vi "GE 1.vi"() -> ()   [LabVIEW 2014]
uses:
  <vilib>/LabVIEW Targets/FPGA/cRIO/shared/nicrio_ModuleControls/nicrio_cRIO-9225_DataRatesRing.ctl
  <vilib>/LabVIEW Targets/FPGA/cRIO/shared/nicrio_ModuleControls/nicrio_cRIO-9227_DataRatesRing.ctl
  <vilib>/rvi/FXPMathLib/FxpSinAndCos/subVIs/nifxpmath_SinAndCos_SimConfig.ctl
  <vilib>/rvi/FXPMathLib/FxpRectToPolar/subVIs/nifxpmath_RectToPolar_SimConfig.ctl
  <vilib>/rvi/FXPMathLib/FxpDiv/subVIs/nifxpmath_Div_SimConfig.ctl
  <vilib>/rvi/Emulation/niFpgaGetClockAttributes.vi
  <vilib>/rvi/Emulation/niFpgaSctlEmulationGetInTimedLoop.vi
  <vilib>/rvi/Emulation/niFpgaEmulationReportErrorSimple.vi
  <vilib>/rvi/eio/common/nirviEmuTemplateMethod_errors.vi
  <vilib>/rvi/Memory/Memory_Emulation/nirvimemoryFastEmulation.vi
  <vilib>/rvi/Memory/Memory_Emulation/nirvimemoryEmulation.vi
  <vilib>/rvi/Emulation/niFpgaEmulationIsFPGAContextNoSignature.vi
  <vilib>/rvi/DataTransferAndStorage/Container/Common/niFpgaContainerGetUniqueNameForEmu.vi
  <vilib>/rvi/Emulation/niFpgaProcessEmulError.vi
  <vilib>/rvi/errors/nirviReportUnexpectedCaseInternalError (U32).vi
  <vilib>/rvi/FXPMathLib/FxpSinAndCos/simVIs/DllFxpSinAndCosTemp_sub.vi
  <vilib>/rvi/FXPMathLib/FxpRectToPolar/simVIs/DllFxpRectToPolarTemp_sub.vi
  <vilib>/rvi/FXPMathLib/FxpDiv/simVIs/DllFxpDivTemp_sub.vi
  <vilib>/rvi/Emulation/niFpgaCriticalErrorInLSC.vi
  <vilib>/rvi/DataTransferAndStorage/Container/Common/niFpgaContainerSetEmuInfo.vi
  <vilib>/rvi/eio/common/nirviEmuReportErrorAndStop.vi
  <vilib>/rvi/eio/common/nirviEmuTemplatePropertySet_noerrors.vi
  <vilib>/eio/EIONode/EIONode.xnode
  <vilib>/rvi/DataTransferAndStorage/Container/XNode/niFpgaContainer.xnode
  <vilib>/rvi/FXPMathLib/FxpSub/XNode/nifxpmath_Sub.xnode
  <vilib>/rvi/FXPMathLib/FxpMul/XNode/nifxpmath_Multiplier.xnode
  <vilib>/rvi/FXPMathLib/FxpSinAndCos/XNode/nifxpmath_SinAndCos.xnode
  <vilib>/rvi/FXPMathLib/FxpAdd/XNode/nifxpmath_Add.xnode
  <vilib>/rvi/FXPMathLib/FxpRectToPolar/XNode/nifxpmath_RectToPolar.xnode
  <vilib>/rvi/FXPMathLib/FxpDiv/XNode/nifxpmath_Div.xnode
  <vilib>/rvi/LocalResourceManager/LocalResourceManager.xnode
  <vilib>/eio/EIOPropertyNode/EIOPropertyNode.xnode
  <vilib>/rvi/eio/common/nirviEmuTemplatePropertyGet_errors.vi
  <vilib>/rvi/eio/common/nirviEmuTemplatePropertyGet_noerrors.vi
  <vilib>/rvi/eio/common/nirviEmuTemplatePropertySet_errors.vi
  <vilib>/rvi/FXPMathLib/sim/FxpSim.dll
panel:
  out "Magnitude Actual":fxp<+,52,38>[](array[numeric])
  out "Angle Actual":fxp<+/-,22,10>[](array[numeric])
  out "Ym Angle":fxp<+/-,22,10>[](array[numeric])
  out "Ym Magnitude":fxp<+/-,64,39>[](array[numeric])
  in  "stop":bool
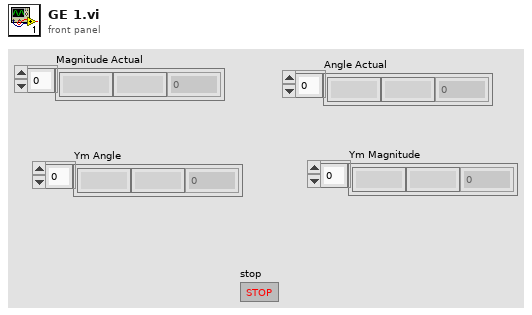
[diagram p1: front panel]
types:
  T1 = typedef "nicrio_cRIO-9227_DataRatesRing.ctl" = u8
  T2 = typedef "nicrio_cRIO-9225_DataRatesRing.ctl" = u8
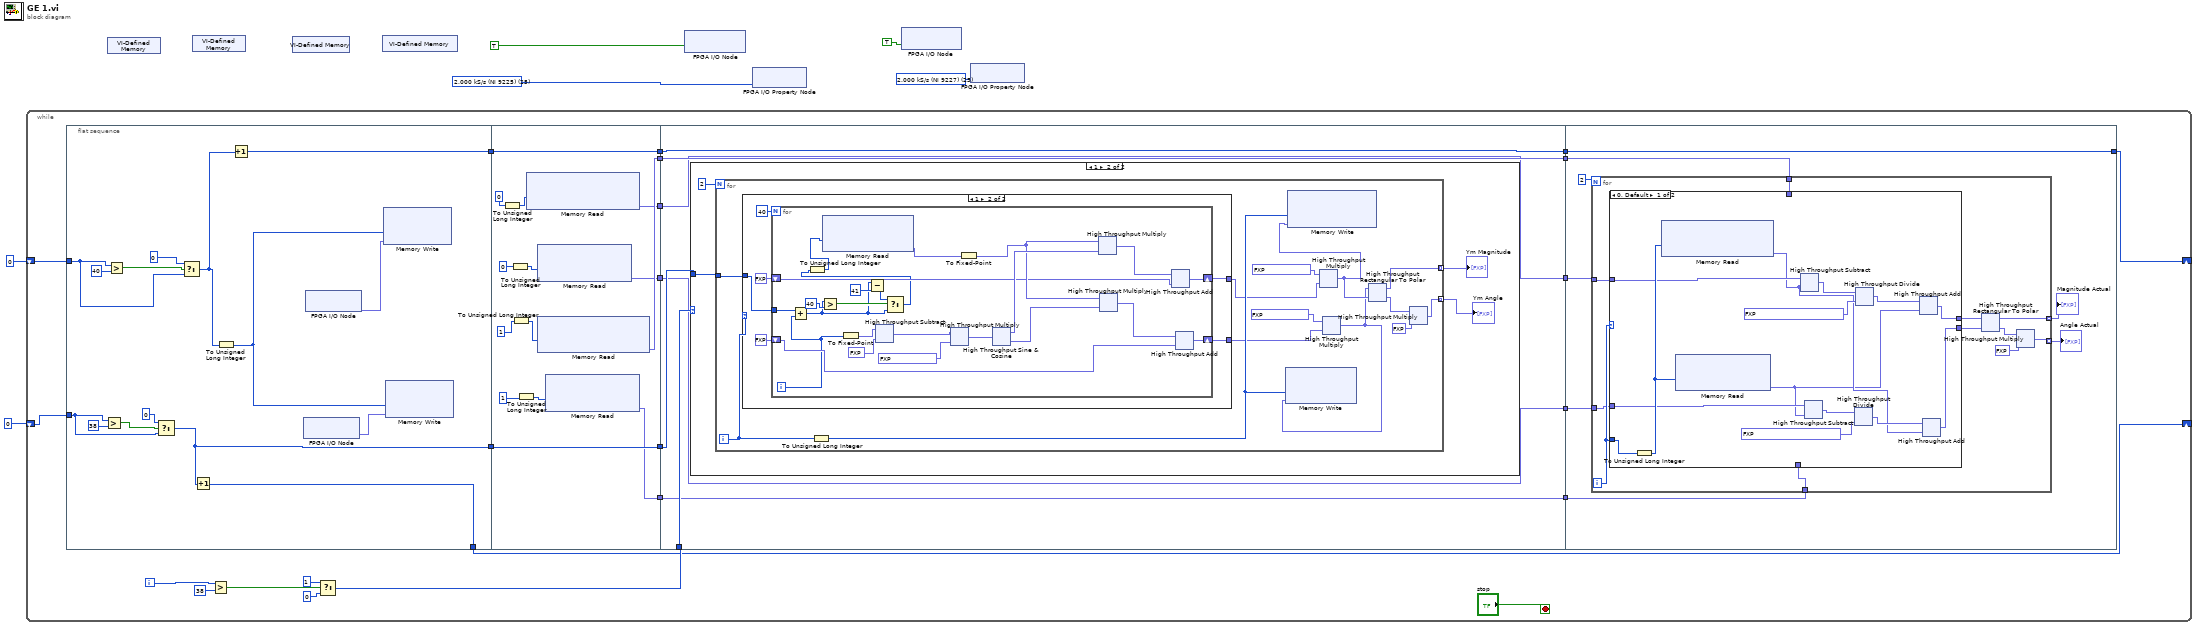
[diagram p0: block diagram]
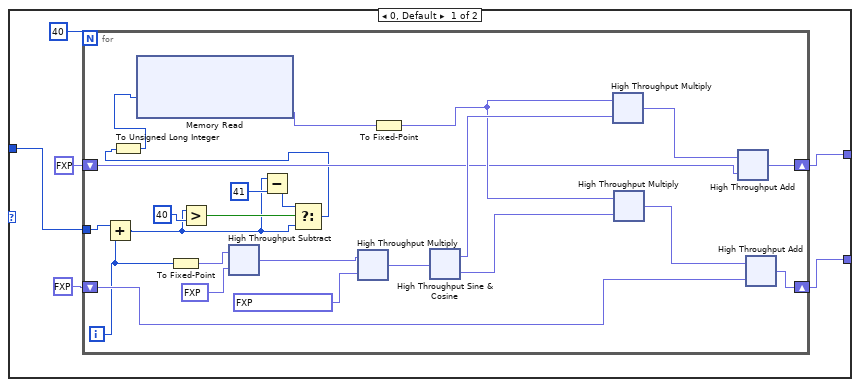
[diagram p3: hidden frame]
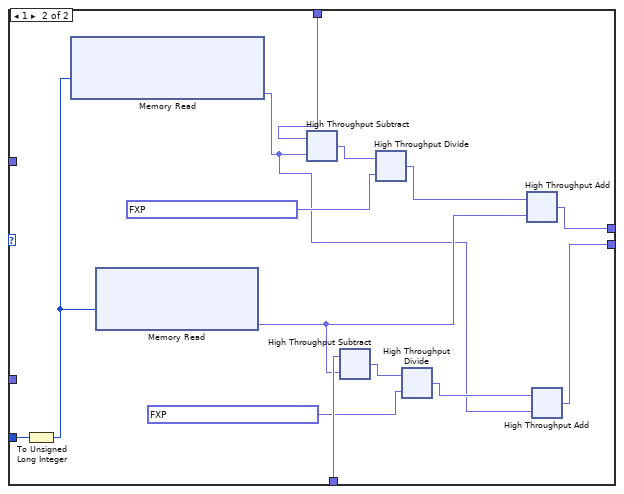
[diagram p4: hidden frame]
diagram:
  w3 = T1 25 items=["50.000 kS/s (NI 9227)"=1, "25.000 kS/s (NI 9227)"=2, "16.667 kS/s (NI 9227)"=3, "12.500 kS/s (NI 9227)"=4, "10.000 kS/s (NI 9227)"=5, "8.333 kS/s (NI 9227)"=6, "7.143 kS/s (NI 9227)"=7, "6.250 kS/s (NI 9227)"=8, "5.556 kS/s (NI 9227)"=9, "5.000 kS/s (NI 9227)"=10, "4.545 kS/s (NI 9227)"=11, "4.167 kS/s (NI 9227)"=12, "3.846 kS/s (NI 9227)"=13, "3.571 kS/s (NI 9227)"=14, "3.333 kS/s (NI 9227)"=15, "3.125 kS/s (NI 9227)"=16, "2.941 kS/s (NI 9227)"=17, "2.778 kS/s (NI 9227)"=18, "2.632 kS/s (NI 9227)"=19, "2.500 kS/s (NI 9227)"=20, "2.381 kS/s (NI 9227)"=21, "2.273 kS/s (NI 9227)"=22, "2.174 kS/s (NI 9227)"=23, "2.083 kS/s (NI 9227)"=24, "2.000 kS/s (NI 9227)"=25, "1.923 kS/s (NI 9227)"=26, "1.852 kS/s (NI 9227)"=27, "1.786 kS/s (NI 9227)"=28, "1.724 kS/s (NI 9227)"=29, "1.667 kS/s (NI 9227)"=30, "1.613 kS/s (NI 9227)"=31] ("Data Rate")
  w4 = T2 25 items=["50.000 kS/s (NI 9225)"=1, "25.000 kS/s (NI 9225)"=2, "16.667 kS/s (NI 9225)"=3, "12.500 kS/s (NI 9225)"=4, "10.000 kS/s (NI 9225)"=5, "8.333 kS/s (NI 9225)"=6, "7.143 kS/s (NI 9225)"=7, "6.250 kS/s (NI 9225)"=8, "5.556 kS/s (NI 9225)"=9, "5.000 kS/s (NI 9225)"=10, "4.545 kS/s (NI 9225)"=11, "4.167 kS/s (NI 9225)"=12, "3.846 kS/s (NI 9225)"=13, "3.571 kS/s (NI 9225)"=14, "3.333 kS/s (NI 9225)"=15, "3.125 kS/s (NI 9225)"=16, "2.941 kS/s (NI 9225)"=17, "2.778 kS/s (NI 9225)"=18, "2.632 kS/s (NI 9225)"=19, "2.500 kS/s (NI 9225)"=20, "2.381 kS/s (NI 9225)"=21, "2.273 kS/s (NI 9225)"=22, "2.174 kS/s (NI 9225)"=23, "2.083 kS/s (NI 9225)"=24, "2.000 kS/s (NI 9225)"=25, "1.923 kS/s (NI 9225)"=26, "1.852 kS/s (NI 9225)"=27, "1.786 kS/s (NI 9225)"=28, "1.724 kS/s (NI 9225)"=29, "1.667 kS/s (NI 9225)"=30, "1.613 kS/s (NI 9225)"=31] ("Data Rate")
  n1 = while {
    shift-right: [w23] -> _
    shift-left: 0 -> [w24]
    shift-right: [w20] -> _
    shift-left: 0 -> [w21]
    i -> [w27]
    stop <- "stop" stop-if-true
    n2 = flat-sequence {
      tunnel: w24 -> [w37]
      tunnel: [w39] -> w18
      tunnel: w21 -> [w33]
      tunnel: [w32] -> w20
      tunnel: [w31] -> w16
      tunnel: w18 -> [w59]
      tunnel: [w59] -> w17
      tunnel: w16 -> [w58]
      tunnel: [w58] -> w15
      tunnel: [w57] -> w13
      tunnel: [w56] -> w11
      tunnel: [w55] -> w9
      tunnel: [w54] -> w7
      tunnel: w25 -> [w66]
      tunnel: w17 -> [w65]
      tunnel: w15 -> [w64]
      tunnel: [w65] -> w19
      tunnel: [w63] -> w14
      tunnel: w13 -> [w63]
      tunnel: [w62] -> w12
      tunnel: w11 -> [w62]
      tunnel: [w61] -> w10
      tunnel: w9 -> [w61]
      tunnel: [w60] -> w8
      tunnel: w7 -> [w60]
      tunnel: [w248] -> w23
      tunnel: w19 -> [w248]
      tunnel: w14 -> [w246]
      tunnel: w12 -> [w245]
      tunnel: w10 -> [w244]
      tunnel: w8 -> [w243]
      frame #0 {
        n3 = Greater?(x=w33, y=38) -> (0:w34:bool)
        n4 = Greater?(x=w37, y=40) -> (0:w44:bool)
        n5 = Select(t=0, s=w34, f=w33) -> (s? t:f=w31:i32)
        n6 = Select(t=0, s=w44, f=w37) -> (s? t:f=w40:i32)
        n7 = Increment(x=w31) -> (x+1=w32:i32)
        n8 = To Unsigned Long Integer(number=w40) -> (unsigned 32bit integer=w43:u32)
        n9 = Increment(x=w40) -> (x+1=w39:i32)
        n10 = xnode "FPGA I/O Node"() -> ("Mod1/AI0"=w42:fxp<+/-,24,10>)  [unwired: 1 in, 1 out]
        n11 = xnode "FPGA I/O Node"() -> ("Mod2/AI0"=w41:fxp<+/-,24,5>)  [unwired: 1 in, 1 out]
        n12 = xnode ("Memory Write")("Address"=w43, "Data"=w41) -> ()  [unwired: 1 in, 1 out]
        n13 = xnode ("Memory Write")("Address"=w43, "Data"=w42) -> ()  [unwired: 1 in, 1 out]
      }
      frame #1 {
        n14 = To Unsigned Long Integer(number=u32 0 ("Address")) -> (unsigned 32bit integer=w52:u32)
        n15 = To Unsigned Long Integer(number=u32 0 ("Address")) -> (unsigned 32bit integer=w50:u32)
        n16 = To Unsigned Long Integer(number=u32 1 ("Address")) -> (unsigned 32bit integer=w48:u32)
        n17 = To Unsigned Long Integer(number=u32 1 ("Address")) -> (unsigned 32bit integer=w46:u32)
        n18 = xnode ("Memory Read")("Address"=w52) -> ("Data"=w55:fxp<+/-,25,11>)  [unwired: 1 in, 1 out]
        n19 = xnode ("Memory Read")("Address"=w50) -> ("Data"=w54:fxp<+/-,25,11>)  [unwired: 1 in, 1 out]
        n20 = xnode ("Memory Read")("Address"=w48) -> ("Data"=w57:fxp<+/-,25,11>)  [unwired: 1 in, 1 out]
        n21 = xnode ("Memory Read")("Address"=w46) -> ("Data"=w56:fxp<+/-,25,11>)  [unwired: 1 in, 1 out]
      }
      frame #2 {
        n22 = case shown="1" w66 {
          tunnel: w64 -> [_ w69]
          frame 0, Default {
          }
          frame 1 {
            n23 = for {
              N: 2 -> [_]
              tunnel: w69 -> [w83]
              tunnel: [w78] -> w68 mode=indexing
              tunnel: [w77] -> w67 mode=indexing
              i -> [w82]
              n24 = case shown="1" w82 {
                tunnel: w83 -> [w123 w183]
                tunnel: [w122 w182] -> w75
                tunnel: [w121 w181] -> w73
                frame 0, Default {
                  n25 = for {
                    N: 40 -> [_]
                    shift-right: [w138] -> w122
                    shift-left: fxp<+/-,64,37> 0.0 ("x+y") -> [w137]
                    shift-right: [w136] -> w121
                    shift-left: fxp<+/-,45,17> 0.0 ("x+y") -> [w135]
                    tunnel: w123 -> [w133]
                    i -> [w134]
                    n26 = Add(x=w133, y=w134) -> (x+y=w127:i32)
                    n27 = To Fixed-Point(number=w134) -> (fixed-point=w150:fxp<+/-,32,32>)  [unwired: 1 in]
                    n28 = Greater?(x=w127, y=40) -> (0:w131:bool)
                    n29 = xnode "High Throughput Subtract"("x"=w150, "y"=fxp<+,6,5> 19.5) -> ("x-y"=w147:fxp<+/-,34,33>)
                    n30 = Subtract(x=w127, y=41) -> (x-y=w129:i32)
                    n31 = Select(t=w129, s=w131, f=w127) -> (s? t:f=w128:i32)
                    n32 = To Unsigned Long Integer(number=w128) -> (unsigned 32bit integer=w141:u32)
                    n33 = xnode ("Memory Read")("Address"=w141) -> ("Data"=w140:fxp<+/-,25,11>)  [unwired: 1 in, 1 out]
                    n34 = xnode ("High Throughput Multiply")("x"=w147, "y"=fxp<+/-,16,1> 0.04998779296875) -> ("x*y"=w146:fxp<+/-,50,34>)
                    n35 = To Fixed-Point(number=w140) -> (fixed-point=w139:fxp<+/-,25,11>)  [unwired: 1 in]
                    n36 = xnode "High Throughput Sine & Cosine"("x (pi)"=w146) -> ("sin(x)"=w145:fxp<+/-,16,2>, "cos(x)"=w144:fxp<+/-,16,2>)
                    n37 = xnode ("High Throughput Multiply")("x"=w139, "y"=w145) -> ("x*y"=w143:fxp<+/-,41,13>)
                    n38 = xnode ("High Throughput Multiply")("x"=w139, "y"=w144) -> ("x*y"=w142:fxp<+/-,41,13>)
                    n39 = xnode ("High Throughput Add")("x"=w143, "y"=w137) -> ("x+y"=w138:fxp<+/-,64,37>)
                    n40 = xnode ("High Throughput Add")("x"=w142, "y"=w135) -> ("x+y"=w136:fxp<+/-,45,17>)
                  }
                }
                frame 1 {
                  n41 = for {
                    N: 40 -> [_]
                    shift-right: [w198] -> w182
                    shift-left: fxp<+/-,64,37> 0.0 ("x+y") -> [w196]
                    shift-right: [w197] -> w181
                    shift-left: fxp<+/-,45,17> 0.0 ("x+y") -> [w195]
                    tunnel: w183 -> [w193]
                    i -> [w194]
                    n42 = Add(x=w193, y=w194) -> (x+y=w188:i32)
                    n43 = Greater?(x=w188, y=40) -> (0:w191:bool)
                    n44 = To Fixed-Point(number=w194) -> (fixed-point=w210:fxp<+/-,32,32>)  [unwired: 1 in]
                    n45 = Subtract(x=w188, y=41) -> (x-y=w189:i32)
                    n46 = xnode "High Throughput Subtract"("x"=w210, "y"=fxp<+,6,5> 19.5) -> ("x-y"=w207:fxp<+/-,34,33>)
                    n47 = Select(t=w189, s=w191, f=w188) -> (s? t:f=w187:i32)
                    n48 = To Unsigned Long Integer(number=w187) -> (unsigned 32bit integer=w201:u32)
                    n49 = xnode ("Memory Read")("Address"=w201) -> ("Data"=w200:fxp<+/-,25,11>)  [unwired: 1 in, 1 out]
                    n50 = xnode ("High Throughput Multiply")("x"=w207, "y"=fxp<+/-,16,1> 0.04998779296875) -> ("x*y"=w206:fxp<+/-,50,34>)
                    n51 = To Fixed-Point(number=w200) -> (fixed-point=w199:fxp<+/-,25,11>)  [unwired: 1 in]
                    n52 = xnode "High Throughput Sine & Cosine"("x (pi)"=w206) -> ("sin(x)"=w205:fxp<+/-,16,2>, "cos(x)"=w204:fxp<+/-,16,2>)
                    n53 = xnode ("High Throughput Multiply")("x"=w199, "y"=w205) -> ("x*y"=w203:fxp<+/-,41,13>)
                    n54 = xnode ("High Throughput Multiply")("x"=w199, "y"=w204) -> ("x*y"=w202:fxp<+/-,41,13>)
                    n55 = xnode ("High Throughput Add")("x"=w203, "y"=w196) -> ("x+y"=w198:fxp<+/-,64,37>)
                    n56 = xnode ("High Throughput Add")("x"=w202, "y"=w195) -> ("x+y"=w197:fxp<+/-,45,17>)
                  }
                }
              }
              n57 = To Unsigned Long Integer(number=w82) -> (unsigned 32bit integer=w81:u32)
              n58 = xnode ("High Throughput Multiply")("x"=fxp<+/-,16,1> 0.03533935546875 ("y"), "y"=w75) -> ("x*y"=w72:fxp<+/-,64,38>)
              n59 = xnode ("Memory Write")("Address"=w81, "Data"=w72) -> ()  [unwired: 1 in, 1 out]
              n60 = xnode ("High Throughput Multiply")("x"=fxp<+/-,16,1> 0.03533935546875 ("y"), "y"=w73) -> ("x*y"=w71:fxp<+/-,61,18>)
              n61 = xnode ("Memory Write")("Address"=w81, "Data"=w71) -> ()  [unwired: 1 in, 1 out]
              n62 = xnode "High Throughput Rectangular To Polar"("x"=w71, "y"=w72) -> ("magnitude"=w77:fxp<+,64,38>, "phase (pi)"=w79:fxp<+/-,16,2>)
              n63 = xnode ("High Throughput Multiply")("x"=w79, "y"=fxp<+,6,8> 180.0) -> ("x*y"=w78:fxp<+/-,22,10>)
            }
            "Ym Magnitude" <- w67
            "Ym Angle" <- w68
          }
        }
      }
      frame #3 {
        n64 = for {
          N: 2 -> [_]
          tunnel: w246 -> [w258]
          tunnel: w245 -> [w257]
          tunnel: w244 -> [w256]
          tunnel: w243 -> [w255]
          tunnel: [w250] -> w242 mode=indexing
          tunnel: [w249] -> w241 mode=indexing
          i -> [w259]
          n65 = case shown="0, Default" w259 {
            tunnel: w259 -> [w309 w377]
            tunnel: w258 -> [_ w376]
            tunnel: w257 -> [_ w375]
            tunnel: w256 -> [w308 _]
            tunnel: w255 -> [w307 _]
            tunnel: [w298 w366] -> w254
            tunnel: [w297 w365] -> w253
            frame 0, Default {
              n66 = To Unsigned Long Integer(number=w309) -> (unsigned 32bit integer=w310:u32)
              n67 = xnode ("Memory Read")("Address"=w310) -> ("Data"=w300:fxp<+/-,25,11>)  [unwired: 1 in, 1 out]
              n68 = xnode ("Memory Read")("Address"=w310) -> ("Data"=w299:fxp<+/-,25,11>)  [unwired: 1 in, 1 out]
              n69 = xnode "High Throughput Subtract"("x"=w308, "y"=w300) -> ("x-y"=w304:fxp<+/-,26,12>)
              n70 = xnode "High Throughput Subtract"("x"=w307, "y"=w299) -> ("x-y"=w305:fxp<+/-,26,12>)
              n71 = xnode "High Throughput Divide"("x"=w305, "y"=fxp<+,29,4> 12.514757186174393) -> ("x/y"=w301:fxp<+/-,37,37>)
              n72 = xnode "High Throughput Divide"("x"=w304, "y"=fxp<+,29,4> 12.514757186174393) -> ("x/y"=w302:fxp<+/-,37,37>)
              n73 = xnode ("High Throughput Add")("x"=w302, "y"=w299) -> ("x+y"=w298:fxp<+/-,52,38>)
              n74 = xnode ("High Throughput Add")("x"=w301, "y"=w300) -> ("x+y"=w297:fxp<+/-,52,38>)
            }
            frame 1 {
              n75 = To Unsigned Long Integer(number=w377) -> (unsigned 32bit integer=w378:u32)
              n76 = xnode ("Memory Read")("Address"=w378) -> ("Data"=w367:fxp<+/-,25,11>)  [unwired: 1 in, 1 out]
              n77 = xnode ("Memory Read")("Address"=w378) -> ("Data"=w368:fxp<+/-,25,11>)  [unwired: 1 in, 1 out]
              n78 = xnode "High Throughput Subtract"("x"=w376, "y"=w367) -> ("x-y"=w372:fxp<+/-,26,12>)
              n79 = xnode "High Throughput Subtract"("x"=w375, "y"=w368) -> ("x-y"=w371:fxp<+/-,26,12>)
              n80 = xnode "High Throughput Divide"("x"=w372, "y"=fxp<+,29,4> 12.514757186174393) -> ("x/y"=w370:fxp<+/-,37,37>)
              n81 = xnode "High Throughput Divide"("x"=w371, "y"=fxp<+,29,4> 12.514757186174393) -> ("x/y"=w369:fxp<+/-,37,37>)
              n82 = xnode ("High Throughput Add")("x"=w370, "y"=w368) -> ("x+y"=w366:fxp<+/-,52,38>)
              n83 = xnode ("High Throughput Add")("x"=w369, "y"=w367) -> ("x+y"=w365:fxp<+/-,52,38>)
            }
          }
          n84 = xnode "High Throughput Rectangular To Polar"("x"=w254, "y"=w253) -> ("magnitude"=w249:fxp<+,52,38>, "phase (pi)"=w251:fxp<+/-,16,2>)
          n85 = xnode ("High Throughput Multiply")("x"=w251, "y"=fxp<+,6,8> 180.0) -> ("x*y"=w250:fxp<+/-,22,10>)
        }
        "Angle Actual" <- w242
        "Magnitude Actual" <- w241
      }
    }
    n86 = Greater?(x=w27, y=38) -> (0:w28:bool)
    n87 = Select(t=1, s=w28, f=0) -> (s? t:f=w25:i32)
  }
  n88 = xnode "VI-Defined Memory"() -> ()  [unwired: 1 out]
  n89 = xnode "VI-Defined Memory"() -> ()  [unwired: 1 out]
  n90 = xnode "VI-Defined Memory"() -> ()  [unwired: 1 out]
  n91 = xnode "VI-Defined Memory"() -> ()  [unwired: 1 out]
  n92 = xnode "FPGA I/O Node"("Mod1/Start"=TRUE) -> ()  [unwired: 1 in, 1 out]
  n93 = xnode "FPGA I/O Property Node"("Data Rate"=w4) -> ()  [unwired: 1 in, 1 out]
  n94 = xnode "FPGA I/O Node"("Mod2/Start"=TRUE) -> ()  [unwired: 1 in, 1 out]
  n95 = xnode "FPGA I/O Property Node"("Data Rate"=w3) -> ()  [unwired: 1 in, 1 out]
